vi "example.vi"() -> ()   [LabVIEW 2013]
uses:
  vi modification tool.lvclass
  add method by reference.vi
panel:
  in  "Path":path
  out "error report":errorcluster[](array[cluster])
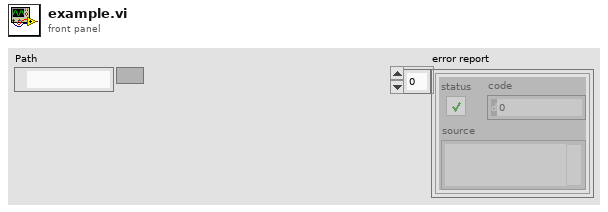
[diagram p1: front panel]
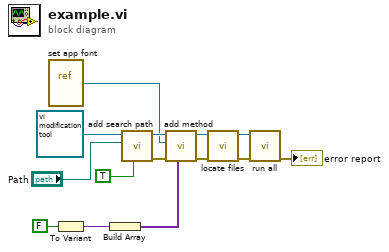
[diagram p0: block diagram]
diagram:
  n1 = vi-ref "set app font.vi"() -> (w4:refnum<vi>)
  n2 = To Variant(anything=FALSE) -> (Variant=w11:variant)
  n3 = Build Array(w11) -> (w2:variant[])
  n4 = call "add search path.vi"("include llb"=TRUE, "Path"="Path", "vi modification tool in"=refnum<class "vi modification tool.lvclass"> refnum ("vi modification tool.lvclass")) -> ("error out"=w3:errorcluster, "vi modification tool out"=w6:refnum<class "vi modification tool.lvclass">)  [unwired: 7 in]
  n5 = call-poly "add method.vi"("parameters"=w2, "error in"=w3, "VI Refnum"=w4, "vi modification tool in"=w6) -> ("error out"=w1:errorcluster, "vi modification tool out"=w5:refnum<class "vi modification tool.lvclass">)  [unwired: 6 in]
  n6 = call "locate files.vi"("error in"=w1, "vi modification tool in"=w5) -> ("error out"=w9:errorcluster, "vi modification tool out"=w10:refnum<class "vi modification tool.lvclass">)  [unwired: 8 in]
  n7 = call "run all.vi"("error in"=w9, "vi modification tool in"=w10) -> ("error report"=→"error report":errorcluster[])  [unwired: 8 in, 1 out]
